vi "DischargeNoRecordingSingleMod.vi"() -> ()   [LabVIEW 2020]
uses:
  <vilib>/addons/NHR/Public/Configure/Output Safety.ctl
  <instrlib>/NH Research Regenerative Test Series/Public/Data/Read (Ave Current).vi
  <instrlib>/NH Research Regenerative Test Series/Public/Data/Low Level/Fetch (Ave Voltage).vi
  <instrlib>/NH Research Regenerative Test Series/Public/Data/Low Level/Fetch (Ave True Power).vi
  <instrlib>/NH Research Regenerative Test Series/NH Research Regenerative Test Series.lvlib
panel:
  out "ErrorOut":string
  in  "Output Safety":T1
  out "Voltage Compare":dbl
  in  "Voltage Cutoff":dbl
  out "Ave Current (A)":dbl
  out "Ave Voltage (V)":dbl
  out "Ave True Power (W)":dbl
  out "Status Byte Register":T2
  in  "Logical Instrument Number":u32=1
  in  "Current Setpoint (0 A)":dbl format="%#.6g"
  in  "Battery Detect Voltage (0V)":dbl format="%#.6g"
  in  "VISA resource name":refnum<visa-resource-name>
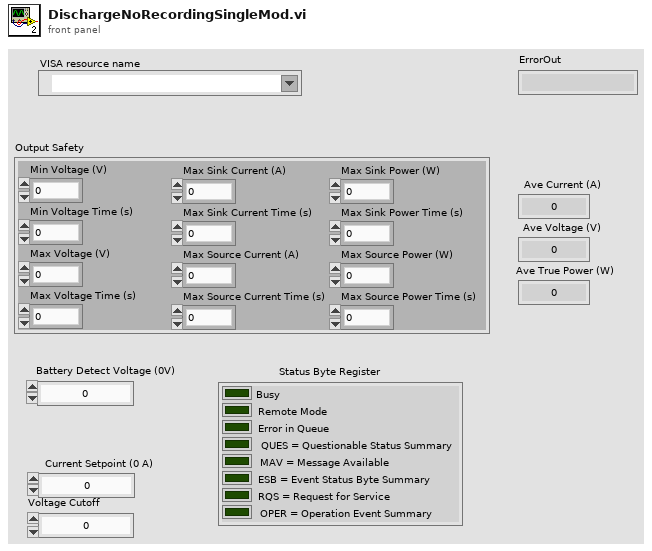
[diagram p1: front panel]
types:
  T1 = typedef "NH Research Regenerative Test Series.lvlib/Output Safety.ctl" = cluster{"Min Voltage (V)":dbl, "Min Voltage Time (s)":dbl, "Max Voltage (V)":dbl, "Max Voltage Time (s)":dbl, "Max Sink Current (A)":dbl, "Max Sink Current Time (s)":dbl, "Max Source Current (A)":dbl, "Max Source Current Time (s)":dbl, "Max Sink Power (W)":dbl, "Max Sink Power Time (s)":dbl, "Max Source Power (W)":dbl, "Max Source Power Time (s)":dbl}
  T2 = cluster{"Busy":bool, "Remote Mode":bool, "Error in Queue":bool, "QUES = Questionable Status Summary":bool, "MAV = Message Available":bool, "ESB = Event Status Byte Summary":bool, "RQS = Request for Service":bool, "OPER = Operation Event Summary":bool}
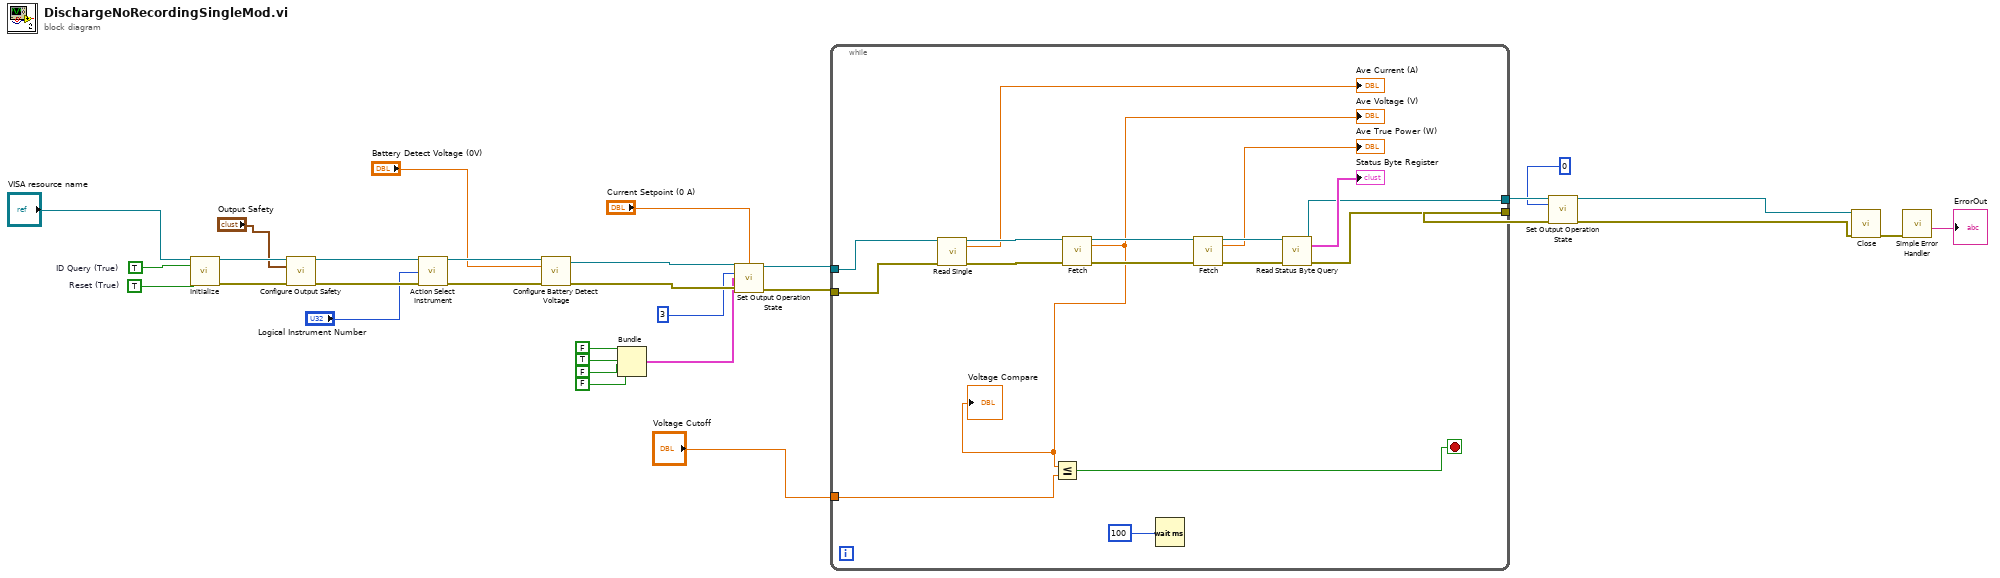
[diagram p0: block diagram]
diagram:
  w15 = TRUE  # ID Query (True)
  w14 = TRUE  # Reset (True)
  n1 = call <instrlib>:"Initialize.vi"("VISA resource name"="VISA resource name", "ID Query (True)"=w15, "Reset (True)"=w14) -> ("VISA resource name out"=w13:refnum<visa-resource-name>, "error out"=w12:errorcluster)  [unwired: 11 in]
  n2 = call <instrlib>:"Configure Output Safety.vi"("VISA resource name"=w13, "Output Safety"="Output Safety", "error in (no error)"=w12) -> ("VISA resource name out"=w10:refnum<visa-resource-name>, "error out"=w5:errorcluster)  [unwired: 11 in]
  n3 = call <instrlib>:"Action Select Instrument.vi"("VISA resource name"=w10, "Logical Instrument Number"="Logical Instrument Number", "error in (no error)"=w5) -> ("VISA resource name out"=w31:refnum<visa-resource-name>, "error out"=w30:errorcluster)  [unwired: 11 in]
  n4 = call <instrlib>:"Configure Battery Detect Voltage.vi"("VISA resource name"=w31, "Battery Detect Voltage (0V)"="Battery Detect Voltage (0V)", "error in (no error)"=w30) -> ("VISA resource name out"=w29:refnum<visa-resource-name>, "error out"=w28:errorcluster)  [unwired: 11 in]
  n5 = Bundle(FALSE, TRUE, FALSE, FALSE) -> (w17:cluster{bool, bool, bool, bool})  [unwired: 1 in]
  n6 = call <instrlib>:"Set Output Operation State.vi"("VISA resource name"=w29, "Current Setpoint (0 A)"="Current Setpoint (0 A)", "Mode (0: Off)"=3, "Enable"=w17, "error in (no error)"=w28) -> ("VISA resource name out"=w24:refnum<visa-resource-name>, "error out"=w23:errorcluster)  [unwired: 9 in]
  n7 = while {
    tunnel: w24 -> [w42]
    tunnel: w23 -> [w41]
    tunnel: [w39] -> w27
    tunnel: [w38] -> w26
    tunnel: "Voltage Cutoff" -> [w35]
    stop <- w36 stop-if-true
    n8 = call-poly <instrlib>:"Read Single.vi"("VISA resource name"=w42, "error in (no error)"=w41) -> ("VISA resource name out"=w47:refnum<visa-resource-name>, "Ave Current (A)"=→"Ave Current (A)":dbl, "error out"=w48:errorcluster)  [unwired: 11 in]
    n9 = call-poly <instrlib>:"Fetch.vi"("VISA resource name"=w47, "error in (no error)"=w48) -> ("VISA resource name out"=w46:refnum<visa-resource-name>, "Ave Voltage (V)"=w32:dbl, "error out"=w45:errorcluster)  [unwired: 11 in]
    "Ave Voltage (V)" <- w32
    "Voltage Compare" <- w32
    n10 = Less Or Equal?(x=w32, y=w35) -> (x <= y?=w36:bool)
    n11 = Wait (ms)(milliseconds to wait=100) -> ()  [unwired: 1 out]
    n12 = call-poly <instrlib>:"Fetch.vi"("VISA resource name"=w46, "error in (no error)"=w45) -> ("VISA resource name out"=w44:refnum<visa-resource-name>, "Ave True Power (W)"=→"Ave True Power (W)":dbl, "error out"=w43:errorcluster)  [unwired: 11 in]
    n13 = call <instrlib>:"Read Status Byte Query.vi"("VISA resource name"=w44, "error in (no error)"=w43) -> ("VISA resource name out"=w39:refnum<visa-resource-name>, "Status Byte Register"=→"Status Byte Register":T2, "error out"=w38:errorcluster)  [unwired: 11 in]
  }
  n14 = call <instrlib>:"Set Output Operation State.vi"("VISA resource name"=w27, "Mode (0: Off)"=0, "error in (no error)"=w26) -> ("VISA resource name out"=w7:refnum<visa-resource-name>, "error out"=w6:errorcluster)  [unwired: 11 in]
  n15 = call <instrlib>:"Close.vi"("VISA resource name"=w7, "error in (no error)"=w6) -> ("error out"=w8:errorcluster)  [unwired: 13 in]
  n16 = call <vilib>:"Simple Error Handler.vi"("error in (no error)"=w8) -> ("source out"=→"ErrorOut":string)  [unwired: 4 in, 4 out]
